vi "Cleanup.vi"(8 "error in (no error)":errorcluster, 11 "VolatusConfig in":refnum<class "VolatusConfig.lvclass">) -> (0 "error out":errorcluster)   [LabVIEW 2020, in "VolatusConfig.lvlib" / "VolatusConfig.lvclass"]
uses:
  VolatusConfig.lvclass
  VolatusConfig.lvclass/VolatusConfig.ctl
  lv-cdm/CDM-Config/Config Manager/Config Manager.lvclass
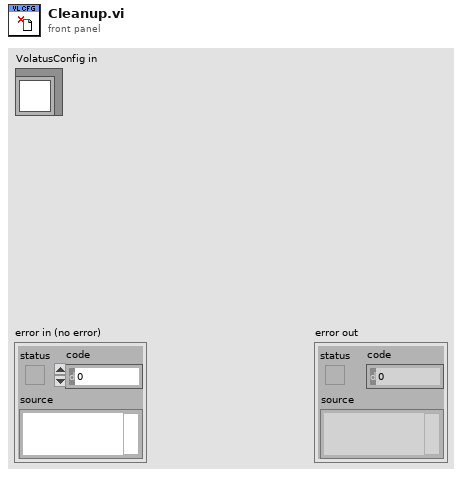
[diagram p1: front panel]
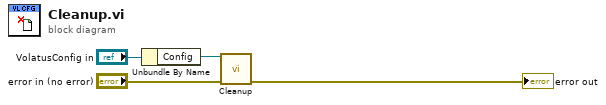
[diagram p0: block diagram]
diagram:
  n1 = Unbundle By Name("VolatusConfig in") -> ("Config"=w2:refnum<class "Config Manager.lvclass">)
  n2 = call "Cleanup.vi"("error in (no error)"="error in (no error)", "Config Manager in"=w2) -> ("error out"=→"error out":errorcluster)  [unwired: 9 in]
